vi "Script Subscribe To Broadcast.vi"(8 "error in (no error)":errorcluster, 9 "Event Name":string="Launch", 11 "Paths":T1={"Target Class"=path "C:/Users/mchi5jm2/LabVIEW/Asynchronous Event Driven Actors/Tooling/Trash/Actor/Message-Enqueuer References.ctl", "API-Reference TD"=path "C:/Users/mchi5jm2/LabVIEW/Asynchronous Event Driven Actors/Tooling/Scripting/Actor/Subscribe to Broadcast.vi"}) -> (0 "error out":errorcluster)   [LabVIEW 2018, in "Scripting.lvlib"]
uses:
  Scripting.lvlib
  Subscribe To Broadcast Component Paths.ctl
  <vilib>/Utility/traverseref.llb/TRef TravTarget.ctl
  <vilib>/Utility/miscctls.llb/LVPositionTypeDef.ctl
  <vilib>/Utility/traverseref.llb/VI Scripting - Traverse.lvlib
  Actor.lvclass
panel:
  in  "VI Save Directory":path
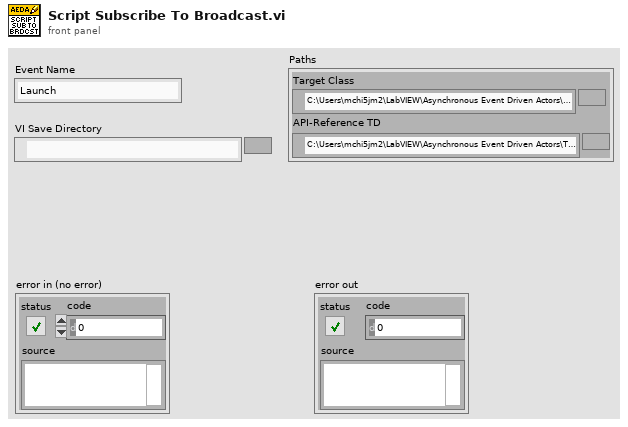
[diagram p1: front panel]
types:
  T1 = typedef "Scripting.lvlib/Subscribe To Broadcast Component Paths.ctl" = cluster{"Target Class":path, "API-Reference TD":path}
  T2 = cluster{"VI":refnum<vi>, "Reg Indicator":refnum<vi>}
  T3 = typedef "TRef TravTarget.ctl" = enum16{"FP", "BD", "Other"}
  T4 = typedef "LVPositionTypeDef.ctl" = cluster{"Left":i32, "Top":i32}
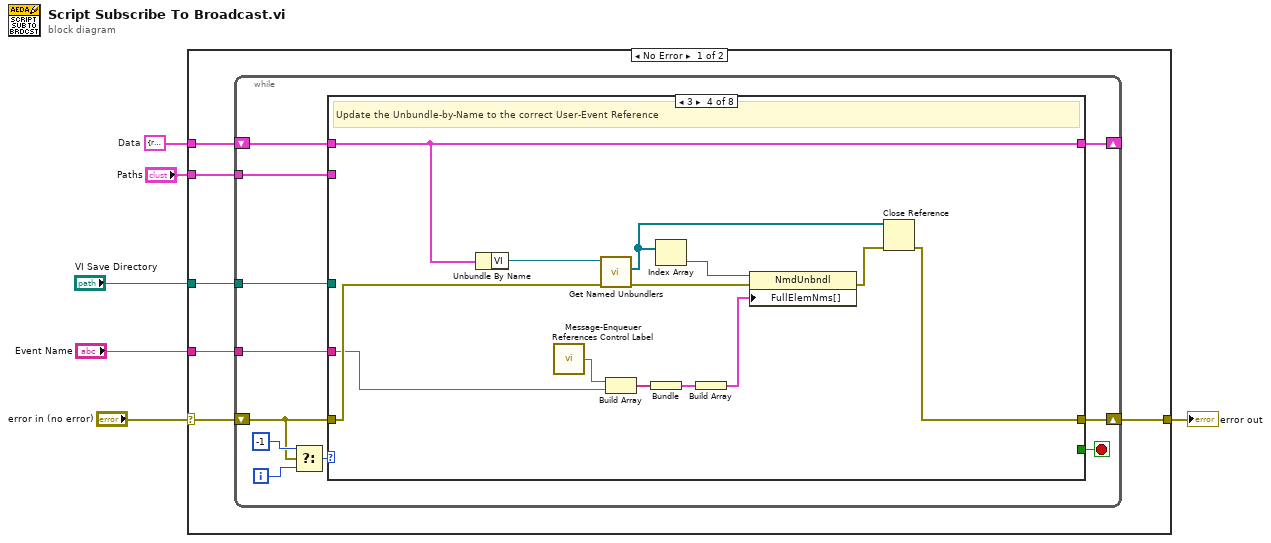
[diagram p0: block diagram]
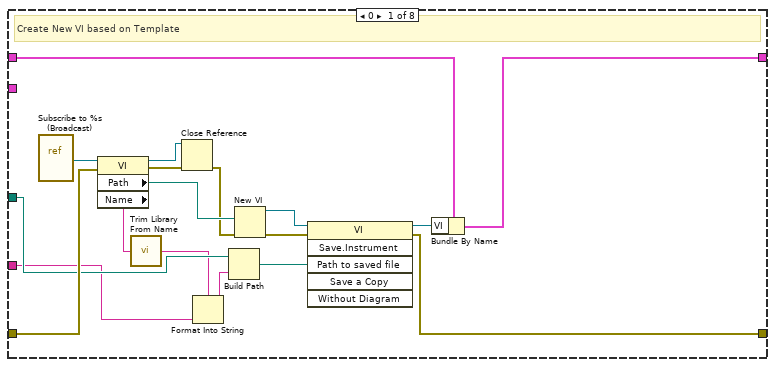
[diagram p2: hidden frame]
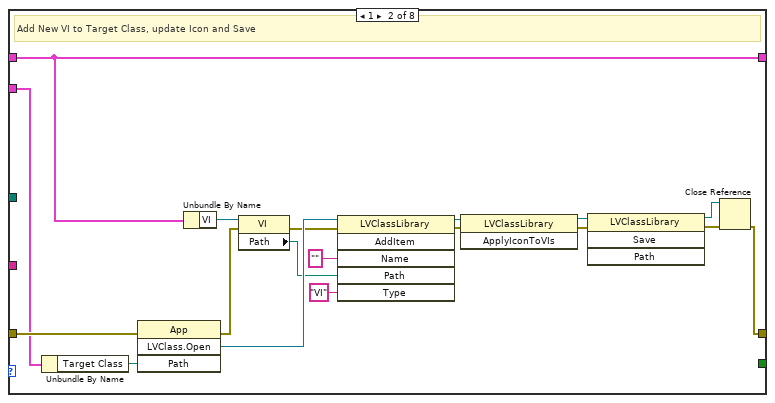
[diagram p3: hidden frame]
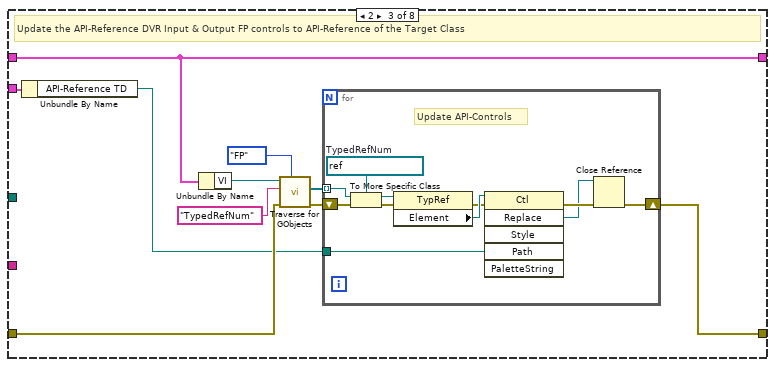
[diagram p4: hidden frame]
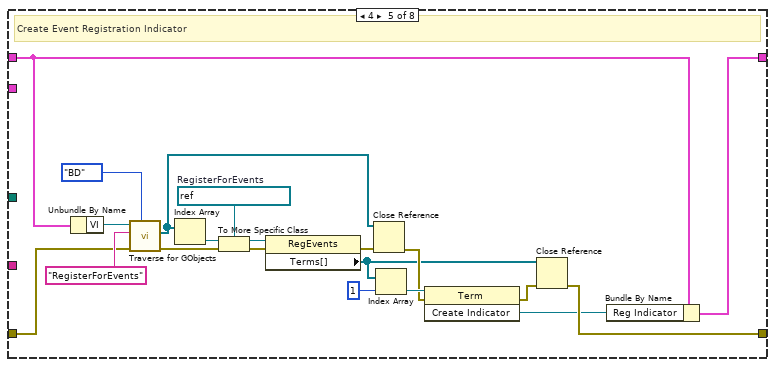
[diagram p5: hidden frame]
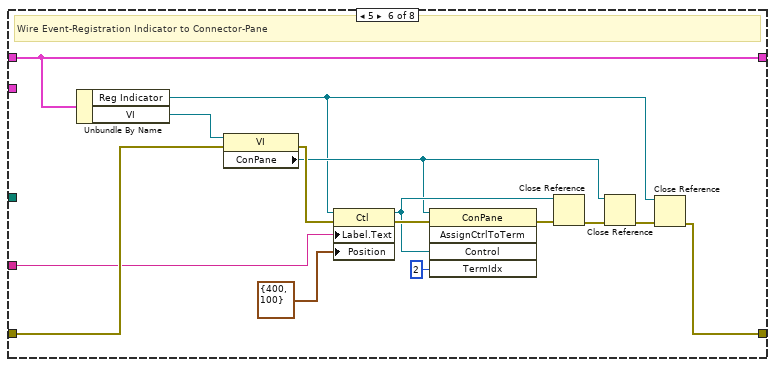
[diagram p6: hidden frame]
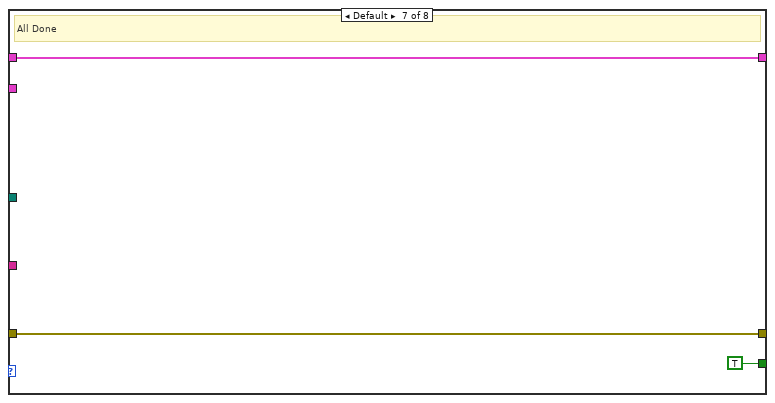
[diagram p7: hidden frame]
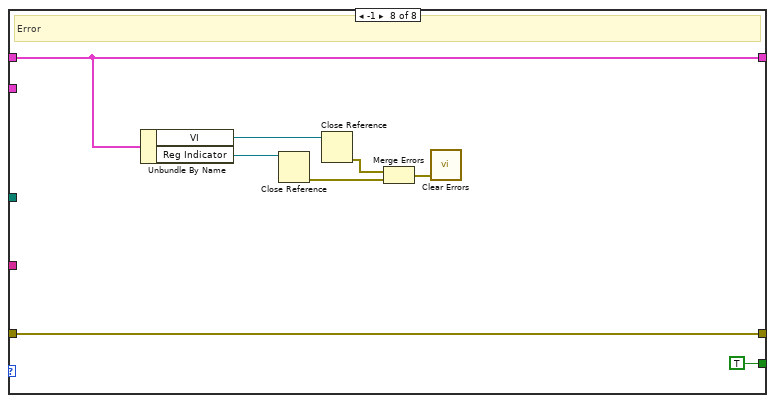
[diagram p8: hidden frame]
diagram:
  w4 = T2 {"VI"=refnum, "Reg Indicator"=refnum}  # Data
  n1 = case shown="No Error" "error in (no error)" {
    selector: "error in (no error)" -> [w12 w140]
    tunnel: "Paths" -> [w11 _]
    tunnel: w4 -> [w10 _]
    tunnel: "Event Name" -> [w9 _]
    tunnel: [w8 w140] -> w2
    tunnel: "VI Save Directory" -> [w7 _]
    frame No Error {
      n2 = while {
        shift-right: [w19] -> w8
        shift-left: w12 -> [w20]
        tunnel: w11 -> [w17]
        shift-right: [w15] -> _
        shift-left: w10 -> [w16]
        tunnel: w9 -> [w14]
        tunnel: w7 -> [w13]
        i -> [w22]
        stop <- w18 stop-if-true
        n3 = Select(t=-1, s=w20, f=w22) -> (s? t:f=w23:i32)
        n4 = case shown="3" w23 {
          tunnel: w20 -> [w33 w59 w65 w88 w109 w127 w131 w138]
          tunnel: [w38 w47 w60 w83 w98 w114 w131 w138] -> w19
          tunnel: [_ _ _ _ _ _ TRUE TRUE] -> w18
          tunnel: w17 -> [_ w58 w64 _ _ _ _ _]
          tunnel: w16 -> [w37 w46 w62 w87 w108 w128 w129 w137]
          tunnel: [w35 w46 w62 w87 w95 w128 w129 w137] -> w15
          tunnel: w14 -> [w25 _ _ w85 _ w121 _ _]
          tunnel: w13 -> [w27 _ _ _ _ _ _ _]
          frame 0 {
            # "Create New VI based on Template"
            n5 = vi-ref "Subscribe to %s (Broadcast).vi"() -> (w34:refnum<vi>)
            n6 = property class="VI"(reference=w34, error in=w33) -> (reference out=w31:refnum<vi>, error out=w30:errorcluster, "Path"=w32:path, "Name"=w28:string)
            n7 = call "Trim Library From Name.vi"("Name in"=w28) -> ("Name out"=w26:string)
            n8 = Close Reference(reference=w31, error in (no error)=w30) -> (error out=w29:errorcluster)
            n9 = Format Into String(format string=w26, w25) -> (resulting string=w24:string)  [unwired: 2 in, 1 out]
            n10 = Build Path(base path=w27, name or relative path=w24) -> (appended path=w39:path)
            n11 = New VI(8:w29, 10:w32) -> (0:w40:errorcluster, 3:w41:refnum<vi>)  [unwired: 5 in]
            n12 = invoke class="VI" method="Save.Instrument"(reference=w41, error in=w40, "Path to saved file"=w39) -> (reference out=w36:refnum<vi>, error out=w38:errorcluster)  [unwired: 3 in, 4 out]
            n13 = Bundle By Name(cluster=w37, "VI"=w36) -> (w35:T2)
          }
          frame 1 {
            # "Add New VI to Target Class, update Icon and Save"
            n14 = Unbundle By Name(w58) -> ("Target Class"=w57:path)
            n15 = invoke class="App" method="LVClass.Open"(error in=w59, "Path"=w57) -> (error out=w43:errorcluster, "LVClass.Open"=w56:refnum<vi>)  [unwired: 2 in, 2 out]
            n16 = Unbundle By Name(w46) -> ("VI"=w45:refnum<vi>)
            n17 = property class="VI"(reference=w45, error in=w43) -> (error out=w42:errorcluster, "Path"=w44:path)  [unwired: 1 out]
            n18 = invoke class="LVClassLibrary" method="AddItem"(reference=w56, error in=w42, "Name"="", "Path"=w44, "Type"="VI") -> (reference out=w53:refnum<vi>, error out=w52:errorcluster)  [unwired: 1 in, 4 out]
            n19 = invoke class="LVClassLibrary" method="ApplyIconToVIs"(reference=w53, error in=w52) -> (reference out=w51:refnum<vi>, error out=w50:errorcluster)  [unwired: 1 in, 1 out]
            n20 = invoke class="LVClassLibrary" method="Save"(reference=w51, error in=w50) -> (reference out=w48:refnum<vi>, error out=w49:errorcluster)  [unwired: 2 in, 2 out]
            n21 = Close Reference(reference=w48, error in (no error)=w49) -> (error out=w47:errorcluster)
          }
          frame 2 {
            # "Update the API-Reference DVR Input & Output FP controls to API-Reference of the Target Class"
            n22 = Unbundle By Name(w64) -> ("API-Reference TD"=w63:path)
            n23 = Unbundle By Name(w62) -> ("VI"=w61:refnum<vi>)
            n24 = call <vilib>:"Traverse for GObjects.vi"("Traverse Target"=TRef_TravTarget."FP", "error in (no error)"=w65, "Class Name"="TypedRefNum", "VI Refnum"=w61) -> ("error out"=w69:errorcluster, "References"=w68:refnum<vi>[])  [unwired: 4 in, 2 out]
            n25 = for {
              tunnel: w68 -> [w80] mode=indexing
              shift-right: [w71] -> w60
              shift-left: w69 -> [w78]
              tunnel: w63 -> [w74]
              w73 = refnum<vi> refnum  # TypedRefNum
              # "Update API-Controls"
              n26 = To More Specific Class(target class=w73, reference=w80, error in=w78) -> (specific class reference=w79:refnum<vi>, error out=w77:errorcluster)
              n27 = property class="TypRef"(reference=w79, error in=w77) -> (error out=w75:errorcluster, "Element"=w76:refnum<vi>)  [unwired: 1 out]
              n28 = invoke class="Ctl" method="Replace"(reference=w76, error in=w75, "Path"=w74) -> (error out=w72:errorcluster, "Replace"=w70:refnum<vi>)  [unwired: 3 in, 4 out]
              n29 = Close Reference(reference=w70, error in (no error)=w72) -> (error out=w71:errorcluster)
            }
          }
          frame 3 {
            # "Update the Unbundle-by-Name to the correct User-Event Reference"
            n30 = Unbundle By Name(w87) -> ("VI"=w86:refnum<vi>)
            n31 = call "Message-Enqueuer References Control Label.vi"() -> ("Message-Enqueuer References Control Label"=w89:string)
            n32 = call "Get Named Unbundlers.vi"("error in (no error)"=w88, "VI in"=w86) -> ("error out"=w90:errorcluster, "NamedUnbundlers"=w81:refnum<vi>[])  [unwired: 6 in, 2 out]
            n33 = Build Array(w89, w85) -> (w91:string[])
            n34 = Bundle(w91) -> (w92:cluster{string[]})  [unwired: 1 in]
            n35 = Index Array(array=w81) -> (element=w82:refnum<vi>)  [unwired: 1 in]
            n36 = Build Array(w92) -> (w93:cluster{string[]}[])
            n37 = property class="NmdUnbndl"(reference=w82, error in=w90, "FullElemNms[]"=w93) -> (error out=w84:errorcluster)  [unwired: 1 out]
            n38 = Close Reference(reference=w81, error in (no error)=w84) -> (error out=w83:errorcluster)
          }
          frame 4 {
            w111 = refnum<vi> refnum  # RegisterForEvents
            # "Create Event Registration Indicator"
            n39 = Unbundle By Name(w108) -> ("VI"=w107:refnum<vi>)
            n40 = call <vilib>:"Traverse for GObjects.vi"("Traverse Target"=TRef_TravTarget."BD", "error in (no error)"=w109, "Class Name"="RegisterForEvents", "VI Refnum"=w107) -> ("error out"=w112:errorcluster, "References"=w96:refnum<vi>[])  [unwired: 4 in, 2 out]
            n41 = Index Array(array=w96) -> (element=w113:refnum<vi>)  [unwired: 1 in]
            n42 = To More Specific Class(target class=w111, reference=w113, error in=w112) -> (specific class reference=w103:refnum<vi>, error out=w104:errorcluster)
            n43 = property class="RegEvents"(reference=w103, error in=w104) -> (error out=w102:errorcluster, "Terms[]"=w100:refnum<vi>[])  [unwired: 1 out]
            n44 = Close Reference(reference=w96, error in (no error)=w102) -> (error out=w101:errorcluster)
            n45 = Index Array(array=w100, index=1) -> (element=w106:refnum<vi>)
            n46 = invoke class="Term" method="Create Indicator"(reference=w106, error in=w101) -> (error out=w99:errorcluster, "Create Indicator"=w94:refnum<vi>)  [unwired: 1 in, 1 out]
            n47 = Close Reference(reference=w100, error in (no error)=w99) -> (error out=w98:errorcluster)
            n48 = Bundle By Name(cluster=w108, "Reg Indicator"=w94) -> (w95:T2)
          }
          frame 5 {
            # "Wire Event-Registration Indicator to Connector-Pane"
            n49 = Unbundle By Name(w128) -> ("Reg Indicator"=w115:refnum<vi>, "VI"=w126:refnum<vi>)
            n50 = property class="VI"(reference=w126, error in=w127) -> (error out=w122:errorcluster, "ConPane"=w117:refnum<vi>)  [unwired: 1 out]
            n51 = property class="Ctl"(reference=w115, error in=w122, "Label.Text"=w121, "Position"=T4 {"Left"=400, "Top"=100}) -> (reference out=w119:refnum<vi>, error out=w124:errorcluster)
            n52 = invoke class="ConPane" method="AssignCtrlToTerm"(reference=w117, error in=w124, "Control"=w119, "TermIdx"=u32 2 ("Terminal Index")) -> (error out=w120:errorcluster)  [unwired: 1 in, 4 out]
            n53 = Close Reference(reference=w119, error in (no error)=w120) -> (error out=w118:errorcluster)
            n54 = Close Reference(reference=w117, error in (no error)=w118) -> (error out=w116:errorcluster)
            n55 = Close Reference(reference=w115, error in (no error)=w116) -> (error out=w114:errorcluster)
          }
          frame Default {
            # "All Done"
          }
          frame -1 {
            # "Error"
            n56 = Unbundle By Name(w137) -> ("VI"=w135:refnum<vi>, "Reg Indicator"=w136:refnum<vi>)
            n57 = Close Reference(reference=w136) -> (error out=w133:errorcluster)  [unwired: 1 in]
            n58 = Close Reference(reference=w135) -> (error out=w134:errorcluster)  [unwired: 1 in]
            n59 = Merge Errors(w134, w133) -> (w132:errorcluster)
            n60 = call <vilib>:"Clear Errors.vi"("error in (no error)"=w132) -> ()  [unwired: 5 in, 2 out]
          }
        }
      }
    }
    frame Error {
    }
  }
  "error out" <- w2
